vi "Update_Rem_gas.vi"(2 "Scan Period (s)":dbl format="%.2f", 4 "Gas Remaining in":dbl format="%.3f", 5 "Ch name":string, 6 "Ch names":string[](array[string]), 7 "Present scan array":dbl[](array[numeric]) format="%.2f") -> (0 "Gas Remaining out":dbl format="%.3f", 1 "Comments":string)   [LabVIEW 2010]
uses:
  Anemometry/Anemometry Sub Vis/Globals/Gas_management_global.vi
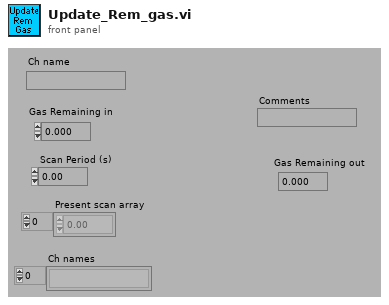
[diagram p1: front panel]
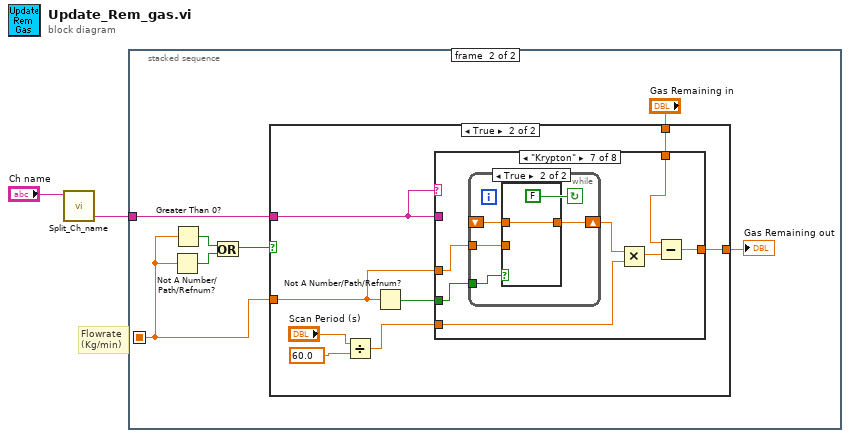
[diagram p0: block diagram]
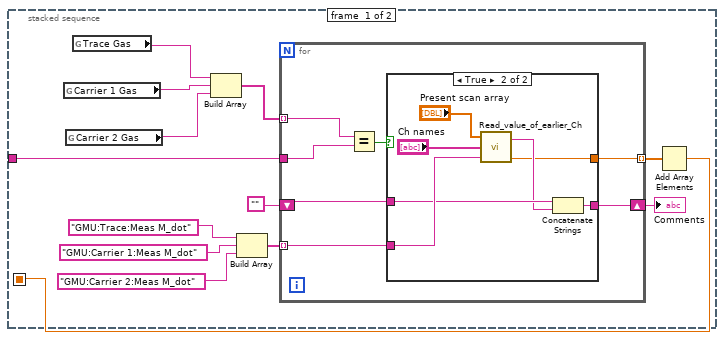
[diagram p2: hidden frame]
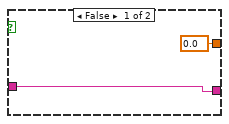
[diagram p3: hidden frame]
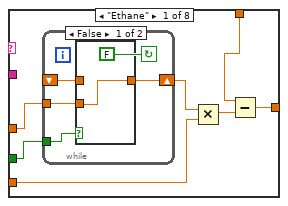
[diagram p5: hidden frame]
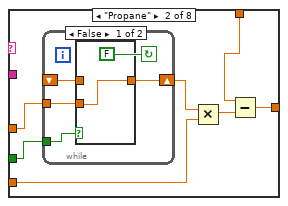
[diagram p7: hidden frame]
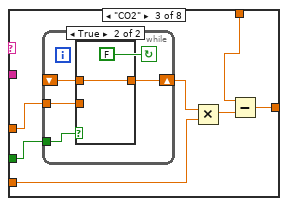
[diagram p9: hidden frame]
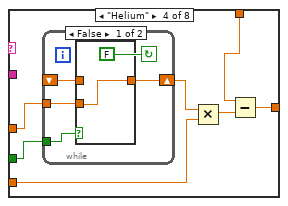
[diagram p11: hidden frame]
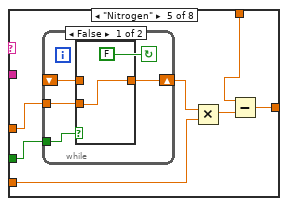
[diagram p13: hidden frame]
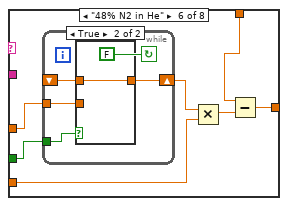
[diagram p15: hidden frame]
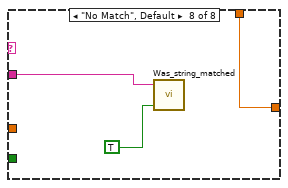
[diagram p18: hidden frame]
diagram:
  # "Flowrate\n(Kg/min)"
  n1 = call "Split_Ch_name.vi"("Ch name"="Ch name") -> ("Low level"=w1:string)  [unwired: 2 out]
  n2 = stacked-sequence {
    seq-local: [w7 _] -> [_ w35]
    tunnel: w1 -> [w10 w36]
    frame #0 {
      n3 = global read "Gas_management_global.vi" "Carrier 1 Gas"() -> (w15:string)
      n4 = global read "Gas_management_global.vi" "Carrier 2 Gas"() -> (w4:string)
      n5 = global read "Gas_management_global.vi" "Trace Gas"() -> (w14:string)
      n6 = Build Array(w14, w15, w4) -> (w11:string[])
      n7 = Build Array("GMU:Trace:Meas M_dot" ("Desired Ch to Read"), "GMU:Carrier 1:Meas M_dot" ("Desired Ch to Read"), "GMU:Carrier 2:Meas M_dot" ("Desired Ch to Read")) -> (w9:string[])
      n8 = for {
        tunnel: w11 -> [w16] mode=indexing
        tunnel: w10 -> [w22]
        tunnel: w9 -> [w20] mode=indexing
        shift-right: [w18] -> w6
        shift-left: "" -> [w19]
        tunnel: [w17] -> w8 mode=indexing
        n9 = Equal?(x=w16, y=w22) -> (x = y?=w21:bool)
        n10 = case shown="True" w21 {
          tunnel: w20 -> [_ w29]
          tunnel: w19 -> [w23 w28]
          tunnel: [w23 w26] -> w18
          tunnel: [0.0 ("Value") w25] -> w17
          frame False {
          }
          frame True {
            n11 = call "Read_value_of_earlier_Ch.vi"("Desired Ch to Read"=w29, "Ch names"="Ch names", "Present scan array"="Present scan array") -> ("Value"=w25:dbl, "Scan comment"=w27:string)  [unwired: 1 in]
            n12 = Concatenate Strings(w28, w27) -> (w26:string)
          }
        }
      }
      "Comments" <- w6
      n13 = Add Array Elements(numeric array=w8) -> (sum=w7:dbl)
    }
    frame #1 {
      n14 = Not A Number/Path/Refnum?(number/path/refnum=w35) -> (NaN/Path/Refnum?=w34:bool)
      n15 = Greater Than 0?(x=w35) -> (x > 0?=w33:bool)
      n16 = Or(x=w33, y=w34) -> (x .or. y?=w32:bool)
      n17 = case shown="True" w32 {
        tunnel: [w39 w44] -> w38
        tunnel: "Gas Remaining in" -> [w39 w43]
        tunnel: w35 -> [_ w41]
        tunnel: w36 -> [_ w40]
        frame False {
        }
        frame True {
          n18 = Divide(x="Scan Period (s)", y=60.0) -> (x/y=w47:dbl)
          n19 = Not A Number/Path/Refnum?(number/path/refnum=w41) -> (NaN/Path/Refnum?=w42:bool)
          n20 = case shown="\"Krypton\"" w40 {
            tunnel: w42 -> [w53 w67 w81 w95 w109 w123 w137 _]
            tunnel: w41 -> [w54 w68 w82 w96 w110 w124 w138 _]
            tunnel: w47 -> [w51 w65 w79 w93 w107 w121 w135 _]
            tunnel: [w49 w63 w77 w91 w105 w118 w132 w148] -> w44
            tunnel: w43 -> [w48 w62 w76 w90 w104 w119 w133 w148]
            tunnel: w40 -> [_ _ _ _ _ _ _ w147]
            frame "Ethane" {
              n21 = while {
                tunnel: w54 -> [w56]
                tunnel: w53 -> [w59]
                shift-left: _ -> [w57]
                shift-right: [w58] -> w50
                stop <- FALSE continue-if-true
                n22 = case shown="False" w59 {
                  tunnel: [w60 w61] -> w58
                  tunnel: w57 -> [_ w61]
                  tunnel: w56 -> [w60 _]
                  frame False {
                  }
                  frame True {
                  }
                }
              }
              n23 = Multiply(x=w50, y=w51) -> (x*y=w52:dbl)
              n24 = Subtract(x=w48, y=w52) -> (x-y=w49:dbl)
            }
            frame "Propane" {
              n25 = while {
                tunnel: w68 -> [w70]
                tunnel: w67 -> [w73]
                shift-left: _ -> [w71]
                shift-right: [w72] -> w64
                stop <- FALSE continue-if-true
                n26 = case shown="False" w73 {
                  tunnel: [w74 w75] -> w72
                  tunnel: w71 -> [_ w75]
                  tunnel: w70 -> [w74 _]
                  frame False {
                  }
                  frame True {
                  }
                }
              }
              n27 = Multiply(x=w64, y=w65) -> (x*y=w66:dbl)
              n28 = Subtract(x=w62, y=w66) -> (x-y=w63:dbl)
            }
            frame "CO2" {
              n29 = while {
                tunnel: w82 -> [w84]
                tunnel: w81 -> [w87]
                shift-left: _ -> [w85]
                shift-right: [w86] -> w78
                stop <- FALSE continue-if-true
                n30 = case shown="True" w87 {
                  tunnel: [w88 w89] -> w86
                  tunnel: w85 -> [_ w89]
                  tunnel: w84 -> [w88 _]
                  frame False {
                  }
                  frame True {
                  }
                }
              }
              n31 = Multiply(x=w78, y=w79) -> (x*y=w80:dbl)
              n32 = Subtract(x=w76, y=w80) -> (x-y=w77:dbl)
            }
            frame "Helium" {
              n33 = while {
                tunnel: w96 -> [w98]
                tunnel: w95 -> [w101]
                shift-left: _ -> [w99]
                shift-right: [w100] -> w92
                stop <- FALSE continue-if-true
                n34 = case shown="False" w101 {
                  tunnel: [w102 w103] -> w100
                  tunnel: w99 -> [_ w103]
                  tunnel: w98 -> [w102 _]
                  frame False {
                  }
                  frame True {
                  }
                }
              }
              n35 = Multiply(x=w92, y=w93) -> (x*y=w94:dbl)
              n36 = Subtract(x=w90, y=w94) -> (x-y=w91:dbl)
            }
            frame "Nitrogen" {
              n37 = while {
                tunnel: w110 -> [w112]
                tunnel: w109 -> [w115]
                shift-left: _ -> [w113]
                shift-right: [w114] -> w106
                stop <- FALSE continue-if-true
                n38 = case shown="False" w115 {
                  tunnel: [w116 w117] -> w114
                  tunnel: w113 -> [_ w117]
                  tunnel: w112 -> [w116 _]
                  frame False {
                  }
                  frame True {
                  }
                }
              }
              n39 = Multiply(x=w106, y=w107) -> (x*y=w108:dbl)
              n40 = Subtract(x=w104, y=w108) -> (x-y=w105:dbl)
            }
            frame "48% N2 in He" {
              n41 = while {
                tunnel: w124 -> [w126]
                tunnel: w123 -> [w129]
                shift-left: _ -> [w127]
                shift-right: [w128] -> w120
                stop <- FALSE continue-if-true
                n42 = case shown="True" w129 {
                  tunnel: [w130 w131] -> w128
                  tunnel: w127 -> [_ w131]
                  tunnel: w126 -> [w130 _]
                  frame False {
                  }
                  frame True {
                  }
                }
              }
              n43 = Multiply(x=w120, y=w121) -> (x*y=w122:dbl)
              n44 = Subtract(x=w119, y=w122) -> (x-y=w118:dbl)
            }
            frame "Krypton" {
              n45 = while {
                tunnel: w138 -> [w140]
                tunnel: w137 -> [w143]
                shift-left: _ -> [w141]
                shift-right: [w142] -> w134
                stop <- FALSE continue-if-true
                n46 = case shown="True" w143 {
                  tunnel: [w144 w145] -> w142
                  tunnel: w141 -> [_ w145]
                  tunnel: w140 -> [w144 _]
                  frame False {
                  }
                  frame True {
                  }
                }
              }
              n47 = Multiply(x=w134, y=w135) -> (x*y=w136:dbl)
              n48 = Subtract(x=w133, y=w136) -> (x-y=w132:dbl)
            }
            frame "No Match", Default {
              n49 = call "Was_string_matched.vi"("Match Error"=TRUE, "Variable name"=w147) -> ()  [unwired: 1 in]
            }
          }
        }
      }
      "Gas Remaining out" <- w38
    }
  }
